vi "Dashboard Main.vi"() -> ()   [LabVIEW 2016]
uses:
  <vilib>/Utility/miscctls.llb/LVRowAndColumnTypeDef.ctl
  <vilib>/event_ctls.llb/eventvkey.ctl
  <vilib>/Rock Robotics/Network Tables/NT Read Numeric Array.vi
  <vilib>/Rock Robotics/WPI/Dashboard/WPI_DashboardLogging Global.vi
panel:
  in  "Camera Settings Right":T1={"Frame Rate"=30, "Compression"=30, "Size"=1, "DB Camera Config"=FALSE} {"Frame Rate" scale=1.0..30.0; "Compression" scale=100.0..-1.0; "Size" items=["640x480", "320x240", "160x120"]}
  in  "Camera Name Right":string(combo)="No Camera Selection"
  out "Camera Info":cluster{"Mbps LED":bool, "Mbps":dbl, "fps":dbl} {"fps" format="%#.1g"; "Mbps" format="%#.1g"}
  in  "Camera Settings":T1={"Frame Rate"=30, "Compression"=30, "Size"=1, "DB Camera Config"=FALSE} {"Frame Rate" scale=1.0..30.0; "Compression" scale=100.0..-1.0; "Size" items=["640x480", "320x240", "160x120"]}
  in  "TCP":refnum<k5>
  in  "Rec Mode":enum32{"Stop", "Record", "Playback"}(radio)
  out "Robot IP":string
  out "Image Message":string="Timeout in Camera Communications"
  in  "Dashboard Tab":T2(tab)
  in  "Select Auto":string(combo)="Select Autonomous ..."
  out "NT Connection":bool
  out "MotorChart R":cluster{"Numeric":dbl, "Numeric":dbl}(graph)
  out "MotorChart L":cluster{"Numeric":dbl, "Numeric":dbl}(graph)
  out "MotorSliders R":cluster{"MotorSlide1":dbl, "MotorSlide2":dbl} {"MotorSlide2" scale=-1.0..1.0 scale format="%#_2e"; "MotorSlide1" scale=-1.0..1.0 scale format="%#_2e"}
  out "MotorSliders L":cluster{"MotorSlide1":dbl, "MotorSlide2":dbl} {"MotorSlide2" scale=-1.0..1.0 scale format="%#_2e"; "MotorSlide1" scale=-1.0..1.0 scale format="%#_2e"}
  out "Gyro":dbl(knob) scale=0.0..360.0
  out "JS1 Z":dbl(slide) scale=-1.0..1.0 scale format="%#_2e"
  out "JS1 Graph":cluster{"X":dbl, "Y":dbl}[](graph)
  out "JS1 Buttons":T3
  out "JS2 Z":dbl(slide) scale=-1.0..1.0 scale format="%#_2e"
  out "JS2 Graph":cluster{"X":dbl, "Y":dbl}[](graph)
  out "JS2 Buttons":T3
  out "Mode":T4(ring)=enum."Auto Disabled"
  out "Camera Image Right":T5(plugin-control)
  in  "DB/String 9":string
  in  "DB/String 8":string
  in  "DB/String 7":string
  in  "DB/String 6":string
  in  "DB/String 5":string
  in  "DB/String 4":string
  in  "DB/String 3":string
  in  "DB/String 2":string
  in  "DB/String 1":string
  in  "DB/String 0":string
  in  "DB/Slider 0":dbl(slide) scale=0.0..5.0
  in  "DB/Slider 1":dbl(slide) scale=0.0..5.0
  in  "DB/Slider 2":dbl(slide) scale=0.0..5.0
  in  "DB/Slider 3":dbl(slide) scale=0.0..5.0
  out "DB/LED 3":bool
  out "DB/LED 2":bool
  out "DB/LED 1":bool
  out "DB/LED 0":bool
  in  "DB/Button 3":bool
  in  "DB/Button 2":bool
  in  "DB/Button 1":bool
  in  "DB/Button 0":bool caption="New Name"
  out "Right Speed":cluster{dbl, dbl}(knob) scale=0.0..3500.0
  out "Left Speed":cluster{dbl, dbl}(knob)={0.0, 1631.277968125847} scale=0.0..3500.0
  out "Right Throttle":dbl
  out "Right Current":dbl
  out "Left Throttle":dbl
  out "Left Current":dbl
  out "Power Consumed":dbl
  out "Voltage":dbl(knob) scale=0.0..14.0
  out "Current Draw":dbl(knob) scale=0.0..300.0
  in  "OSC Stream":bool
  in  "Test Slider":dbl(slide) scale=0.0..100.0 scale format="%#_3g"
  in  "On/Off":bool caption="Solenoid"
  in  "Test Name":u16(ring) items=["Select the test to run..."]
  in  "Test Tree":string(tree)
  in  "Motor":cluster{"Value":dbl, "Enable":bool} {"Value" scale=-1.0..1.0 scale format="%#_3g"}
  out "Progress":T6 {"Test Progress" scale=0.0..100.0}
  in  "Rev/Fwd":cluster{"Forward":bool, "Reverse":bool}
  in  "Test Ring":u16(ring) items=["Monochrome", "Color"]
  out "Cmd Status":string
  in  "Execute Command":bool
  in  "Command Params":string[][](table)
  in  "Command Selection":i32(listbox)
  in  "CheckList":i32(listbox)
  out "Tree":string(tree)
  out "Camera Image":T5(plugin-control)
  out "Background":bool
  in  "Camera Name":string(combo)="No Camera Selection"
  # "HW"
  # "HW"
  # "Joysticks"
  # "Drive Motors"
  # "Front"
  # "Right"
  # "Left"
  # "Back"
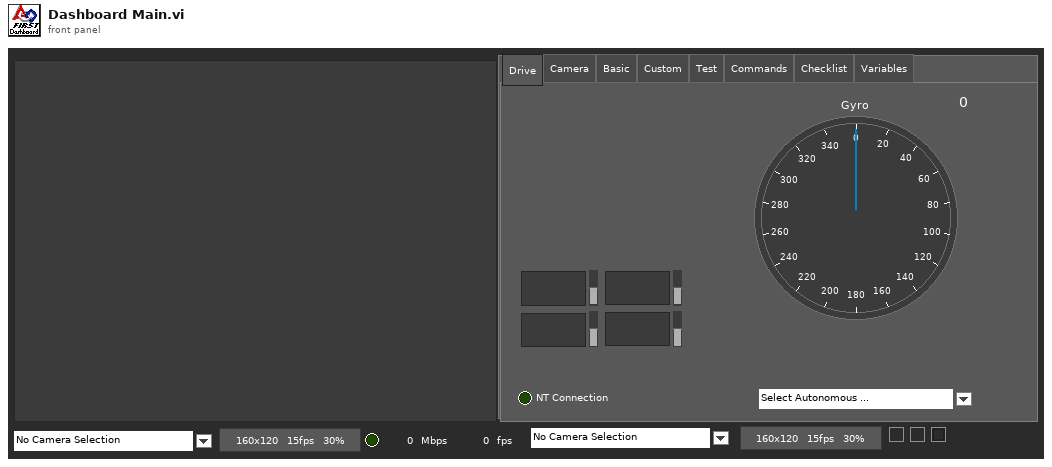
[diagram p1: front panel]
types:
  T1 = cluster{"Frame Rate":i32, "Compression":i32, "Size":u16, "DB Camera Config":bool}
  T2 = enum32{"Drive", "Camera", "Basic", "Custom", "Test", "Commands", "Checklist", "Variables"}
  T3 = cluster{bool, bool, bool, bool, bool, bool, bool, bool, bool, bool, bool, bool}
  T4 = enum8{"Tele-Op Disabled", "Tele-Op Enabled", "Auto Disabled", "Auto Enabled", "Test Disabled", "Test Enabled", "Disconnected", "No Code", "E-Stop"}
  T5 = typedef "IMAQ Image.ctl" = refnum<image>
  T6 = cluster{"Test Progress":u8, "Test Progress Text":string}
  T7 = typedef "Image Type" = u32
  T8 = cluster{"IDs":cluster{"RPC field ID":u16, "Unique ID":u16}, "String":string}
  T9 = enum32{"Drive", "Basic", "Custom", "Test", "Checklist", "Variables"}
  T10 = cluster{"Error Strings":string, "Disable Counts":cluster{u16, u16}, "Rail Faults":cluster{u16, u16, u16}, "Robot IP":string, "DB Mode":u8, "Event Info":cluster{"Name":string, "Type":u8, "Number":u16, "Replay":u8}}
  T11 = cluster{"Storage":cluster{"Disk Free":u64, "RAM Block":u32, "RAM free":u32}, "CPU Utilization":cluster{"CPU % ISR":sgl, "CPU % Time Crit":sgl, "CPU % Timed Str":sgl, "CPU % High":sgl, "CPU % Above":sgl, "CPU % Normal":sgl, "CPU % Low":sgl}, "CAN":cluster{"% Bus Utilization":sgl, "Bus Off Cnt":u32, "TX_FIFO Full Cnt":u32, "Receive Error Cnt":u8, "Transmit Error Cnt":u8}, "HID":cluster{"HID Outputs":u32, "Rumble Low":u16, "Rumble High":u16}[]}
  T12 = cluster{"Status bits":cluster{"Test Mode":bool, "Autonomous":bool, "Enabled":bool, "Code Start":bool, "Brownout":bool, "Reserved 2":bool, "Reserved 3":bool, "E-Stop":bool}, "Code Trace":cluster{"Disabled":bool, "TeleOp":bool, "Auto":bool, "Test":bool}, "Controller Type":enum16{"unknown", "cRIO", "roboRio"}, "Code?":enum16{"unknown", "noCode", "code"}, "Battery V":dbl}
  T13 = cluster{"Control Bits":cluster{"TestMode":bool, "Autonomous":bool, "Enabled":bool, "FMS Present":bool, bool, bool, bool, "E-Stop":bool}, "Team Station ":u8, "Countdown":sgl, "Joystick Values":cluster{"Axes":dbl[], "Buttons":bool[], "POVs":i16[]}[]}
  T14 = cluster{"Axes":dbl[], "Buttons":bool[], "POVs":i16[]}[]
  T15 = cluster{"Axes":dbl[], "Buttons":bool[], "POVs":i16[]}
  T16 = cluster{"Buttons[0]":bool, "Buttons[1]":bool, "Buttons[2]":bool, "Buttons[3]":bool, "Buttons[4]":bool, "Buttons[5]":bool, "Buttons[6]":bool, "Buttons[7]":bool, "Buttons[8]":bool, "Buttons[9]":bool, "Buttons[10]":bool, "Buttons[11]":bool}
  T17 = cluster{"Camera Image":refnum<vi>, "Dashboard Tab":refnum<vi>, "Background":refnum<vi>, "Rec Mode":refnum<vi>, "Test Slider":refnum<vi>, "On/Off ":refnum<vi>, "Test Ring":refnum<vi>, "Rev/Fwd":refnum<vi>, "Test Name":refnum<vi>, "Motor":refnum<vi>, "Progress":refnum<vi>, "CheckList":refnum<vi>, "Tree":refnum<vi>, "Test Tree":refnum<vi>, "Command Params":refnum<vi>, "Command Selection":refnum<vi>, "Execute Command":refnum<vi>, "Cmd Status":refnum<vi>, "Camera Settings":refnum<vi>, "Camera Name":refnum<vi>, "Camera Info":refnum<vi>, "Camera Settings Right":refnum<vi>, "Camera Name Right":refnum<vi>, "Camera Image Right":refnum<vi>}
  T18 = cluster{"Operation":enum16{"Update", "Clear"}, "Color Box":u32}[]
  T19 = typedef "eventvkey.ctl" = enum16{"ASCII", "Enter", "Return", "Shift", "Ctrl", "Alt", "Cmd", "Opt", "Caps", "NumLock", "Clear", "Break", "Up", "Down", "Left", "Right", "Insert", "Delete", "Home", "End", "PageUp", "PageDown", "Escape", "Help", "Pause", "ScrollLock", "F1", "F2", "F3", "F4", "F5", "F6", "F7", "F8", "F9", "F10", "F11", "F12", "F13", "F14", "F15", "F16", "F17", "F18", "F19", "F20", "F21", "F22", "F23", "F24", "Play", "VolumeUp", "VolumeDown", "Mute", "Two Byte Char"}
  T20 = cluster{"Image Size":bool, "Image Type":bool, "Pixel Value":bool, "ROI Information":bool, "Zoom Factor":bool}
  T21 = cluster{"Operation":enum16{"Update", "Clear"}, "Color Box":u32}
  T22 = typedef "LVRowAndColumnTypeDef.ctl" = cluster{"Row":i32, "Column":i32}
  T23 = cluster{"Shift":bool, "Ctrl":bool, "Alt":bool, "Cmd":bool, "Opt":bool}
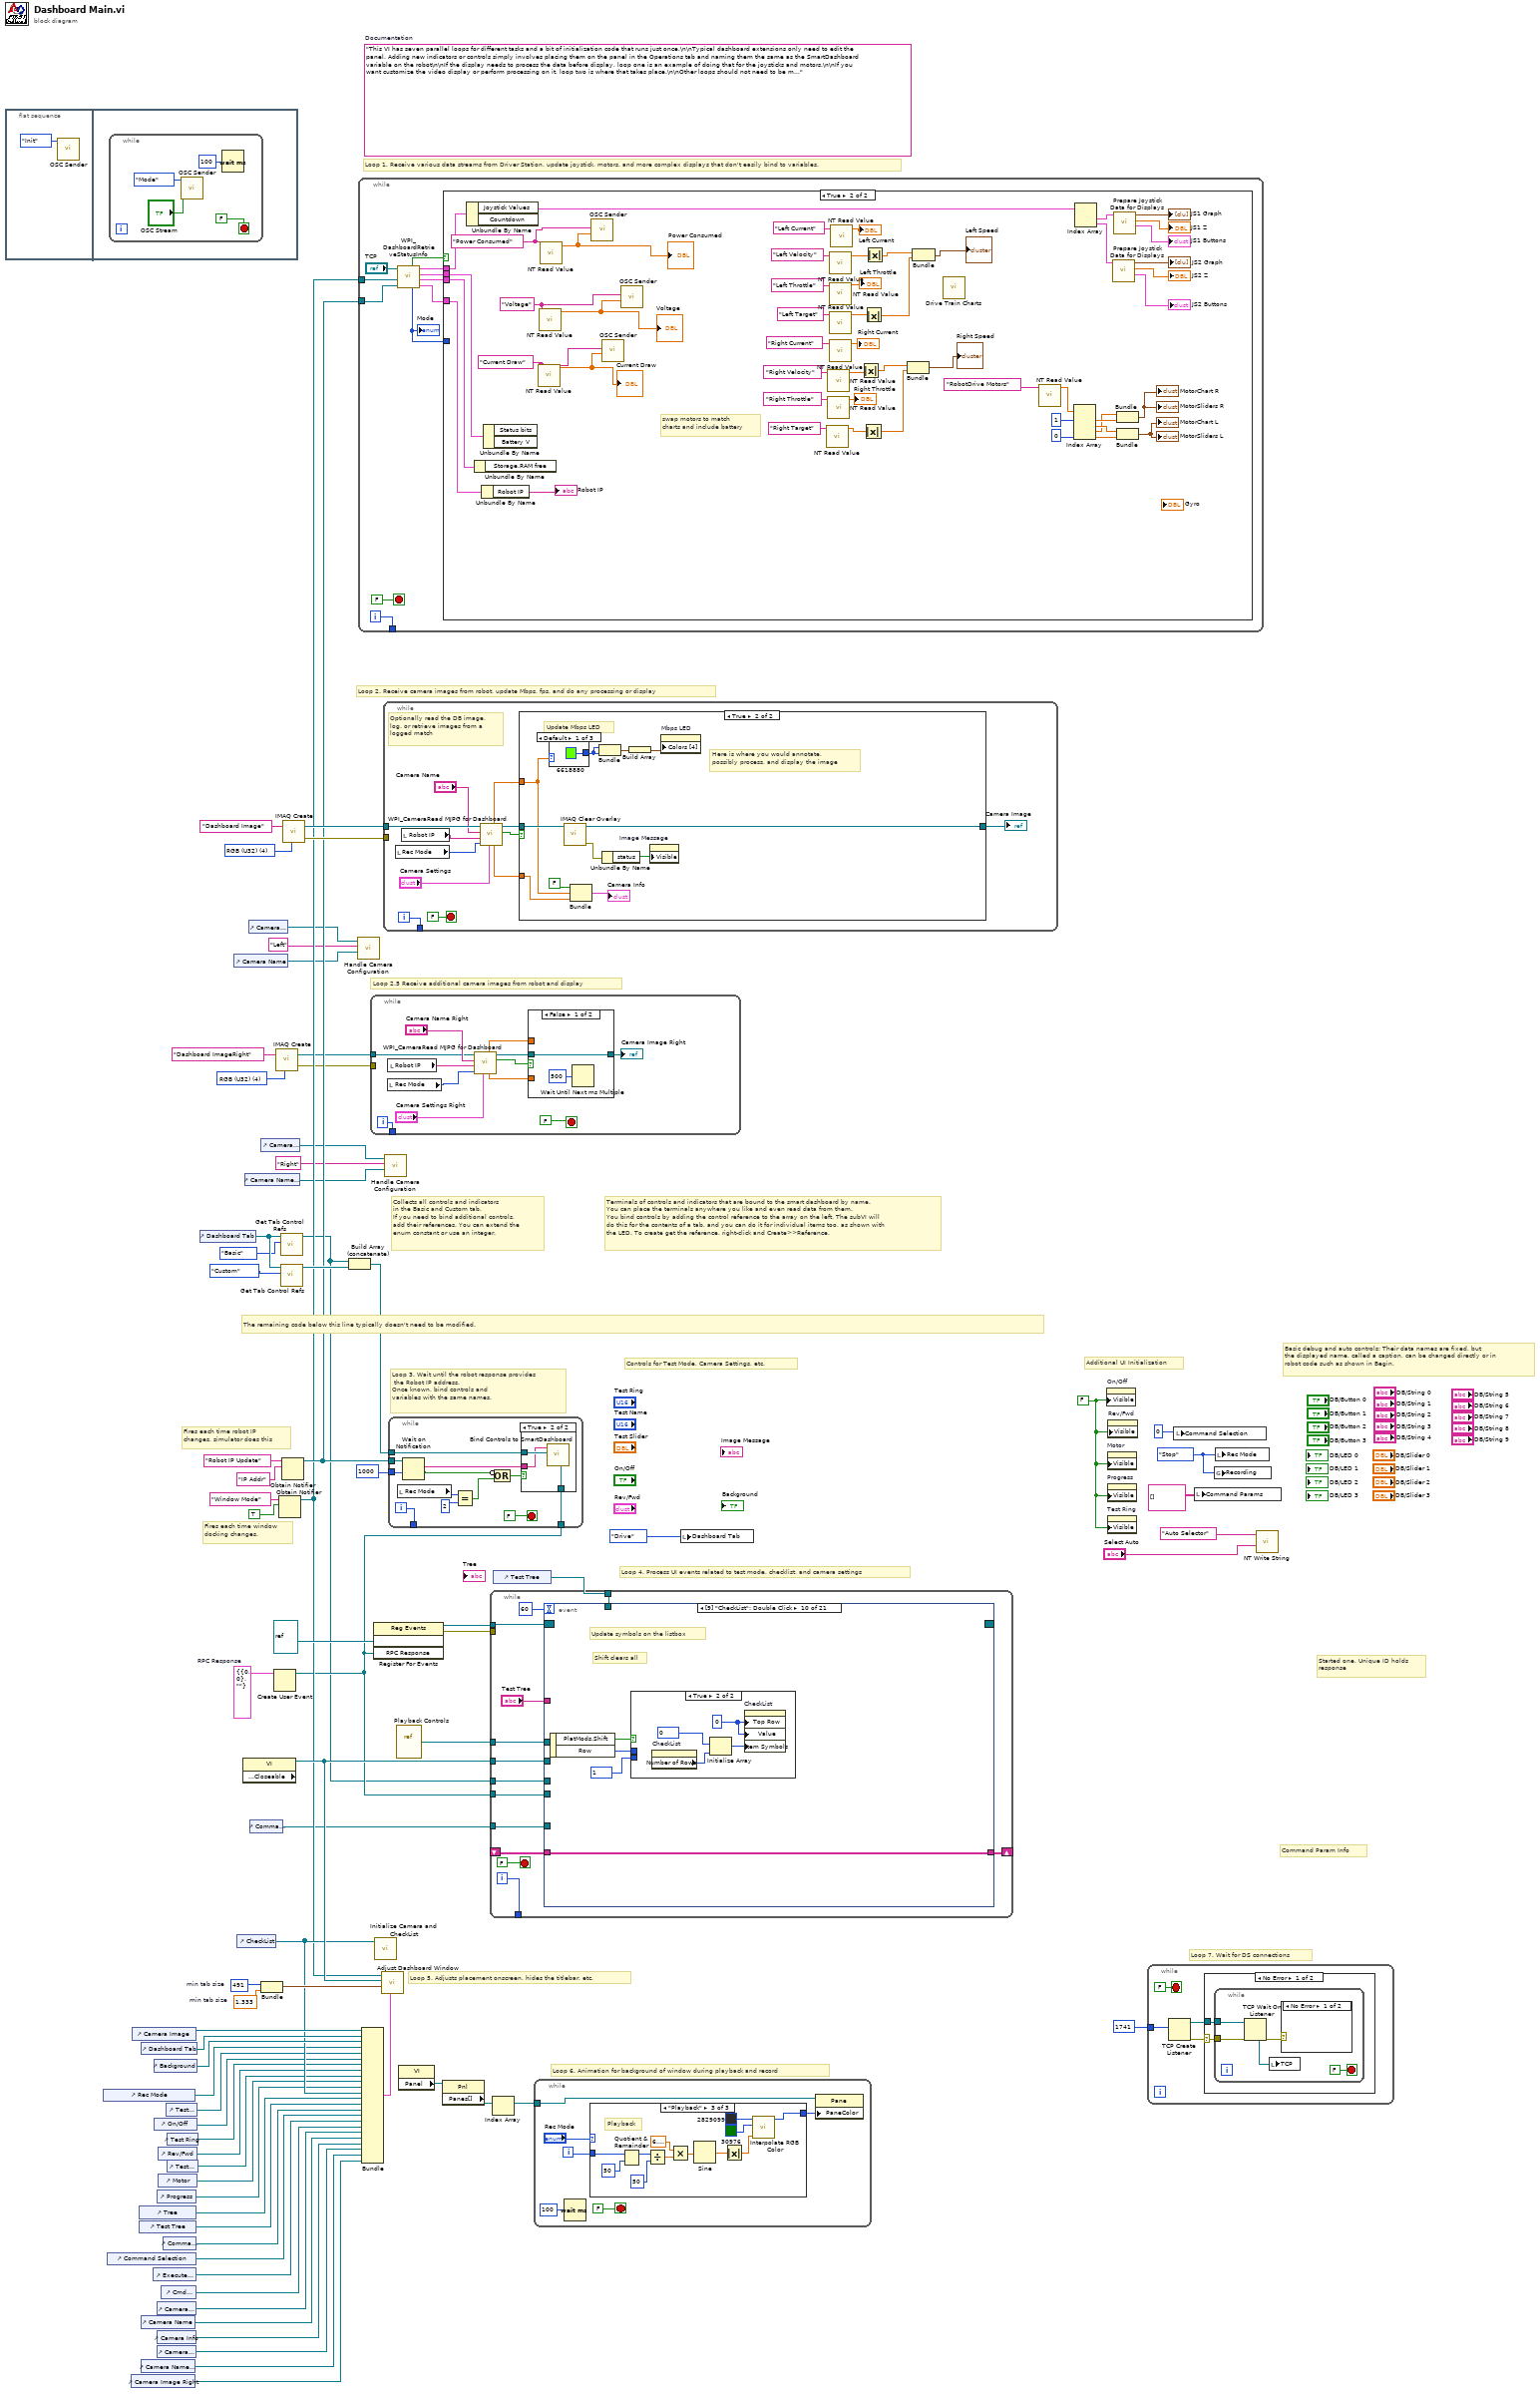
[diagram p0: block diagram]
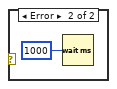
[diagram p3: hidden frame]
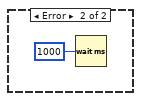
[diagram p4: hidden frame]
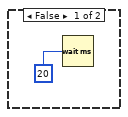
[diagram p5: hidden frame]
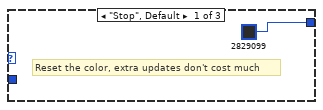
[diagram p6: hidden frame]
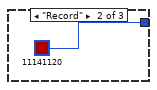
[diagram p7: hidden frame]
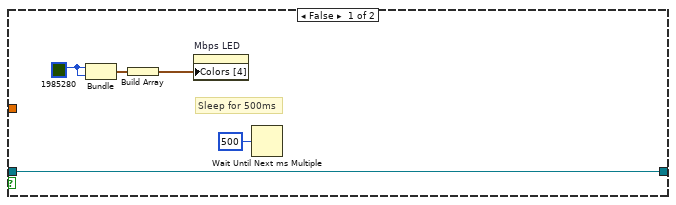
[diagram p9: hidden frame]
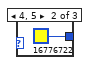
[diagram p10: hidden frame]
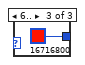
[diagram p11: hidden frame]
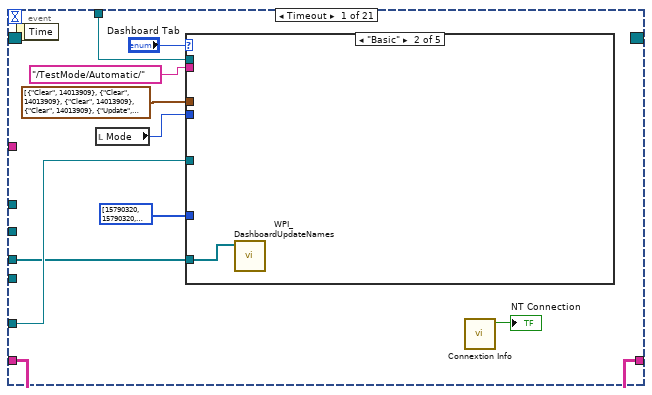
[diagram p12: hidden frame]
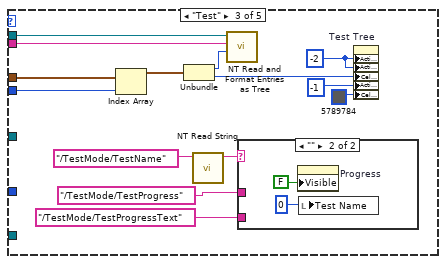
[diagram p14: hidden frame]
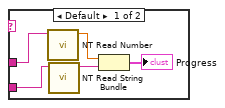
[diagram p15: hidden frame]
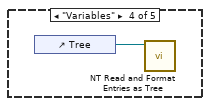
[diagram p16: hidden frame]
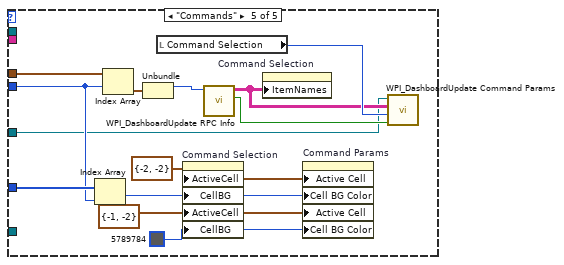
[diagram p17: hidden frame]
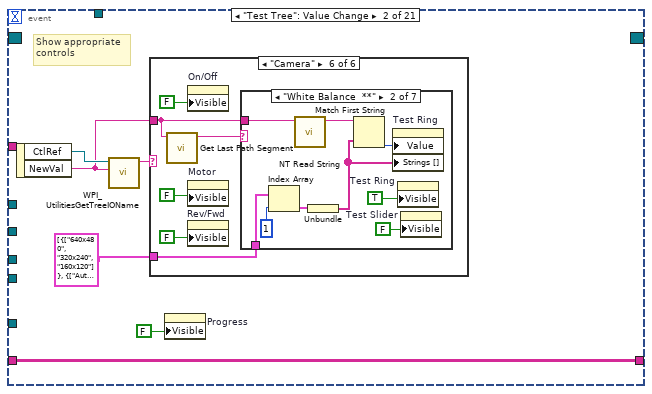
[diagram p18: hidden frame]
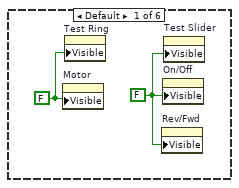
[diagram p19: hidden frame]
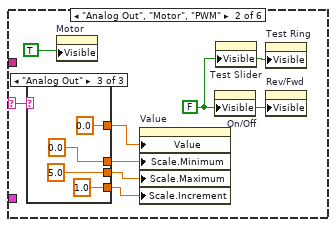
[diagram p20: hidden frame]
diagram:
  w10 = T7 4 items=["Grayscale (U8)", "Grayscale (I16)", "Grayscale (SGL)", "Complex (CSG)", "RGB (U32)", "HSL (U32)", "RGB (U64)"] ("Image Type")
  w26 = T8 {"IDs"={"RPC field ID"=0, "Unique ID"=0}, "String"=""}  # RPC Response
  w51 = 491  # min tab size
  w50 = 1.333  # min tab size
  w58 = enum32{"Stop", "Record", "Playback"}."Stop" ("Rec Mode")
  w33 = FALSE ("Visible")
  (unwired) "This VI has seven parallel loops for different tasks and a bit of initialization code that runs just once.\n\nTypical dashboard extensions only need to edit the panel. Adding new indicators or controls simply involves placing them on the panel in the Operations tab and naming them the same as the SmartDashboard variable on the robot\n\nIf the display needs to process the data before display, loop one is an example of doing that for the joysticks and motors.\n\nIf you want customize the video display or perform processing on it, loop two is where that takes place.\n\nOther loops should not need to be modified. They are pretty standard, and document the task they perform."  # Documentation
  w75 = T7 4 items=["Grayscale (U8)", "Grayscale (I16)", "Grayscale (SGL)", "Complex (CSG)", "RGB (U32)", "HSL (U32)", "RGB (U64)"] ("Image Type")
  # "Loop 2.5 Receive additional camera images from robot and display"
  # "Command Param Info"
  # "Started one, Unique ID holds\nresponse"
  # "Loop 7. Wait for DS connections"
  # "Basic debug and auto controls: Their data names are fixed, but\nthe displayed name, called a caption, can be changed directly or in\nrobot code such as shown in Begin."
  # "Controls for Test Mode, Camera Settings, etc."
  # "Additional UI Initialization"
  # "Loop 6. Animation for background of window during playback and record"
  # "Fires each time robot IP\nchanges, simulator does this"
  # "Fires each time window\ndocking changes."
  # "Collects all controls and indicators\nin the Basic and Custom tab.\nIf you need to bind additional controls,\nadd their references. You can extend the\nenum constant or use an integer."
  # "The remaining code below this line typically doesn't need to be modified."
  # "Loop 4. Process UI events related to test mode, checklist, and camera settings"
  # "Terminals of controls and indicators that are bound to the smart dashboard by name.\nYou can place the terminals anywhere you like and even read data from them.\nYou bind controls by adding the control reference to the array on the left. The subVI will\ndo this for the contents of a tab, and you can do it for individual items too, as shown with\nthe LED. To create get the reference, right-click and Create>>Reference."
  # "Loop 3. Wait until the robot response provides\n the Robot IP address.\nOnce known, bind controls and\nvariables with the same names."
  # "Loop 5. Adjusts placement onscreen, hides the titlebar, etc."
  # "Loop 1. Receive various data streams from Driver Station, update joystick, motors, and more complex displays that don't easily bind to variables."
  # "Loop 2. Receive camera images from robot, update Mbps, fps, and do any processing or display"
  n1 = flat-sequence {
    frame #0 {
      n2 = call "OSC Sender.vi"("State"=enum16{"Init", "Send", "Mode"}."Init") -> ()  [unwired: 11 in]
    }
    frame #1 {
      n3 = while {
        stop <- FALSE stop-if-true
        n4 = call "OSC Sender.vi"("Mode"="OSC Stream", "State"=enum16{"Init", "Send", "Mode"}."Mode") -> ()  [unwired: 10 in]
        n5 = Wait (ms)(milliseconds to wait=u32 100) -> ()  [unwired: 1 out]
      }
    }
  }
  n6 = control-ref of="Rec Mode"() -> (w39:refnum<vi>)
  n7 = control-ref of="Command Selection"() -> (w25:refnum<vi>)
  n8 = control-ref of="Camera Image Right"() -> (w1:refnum<vi>)
  n9 = control-ref of="Camera Image"() -> (w53:refnum<vi>)
  n10 = control-ref of="Tree"() -> (w43:refnum<vi>)
  n11 = control-ref of="Test Tree"() -> (w42:refnum<vi>)
  n12 = control-ref of="Dashboard Tab"() -> (w52:refnum<vi>)
  n13 = control-ref of="Camera Name"() -> (w16:refnum<vi>)
  n14 = control-ref of="Camera Name Right"() -> (w2:refnum<vi>)
  n15 = control-ref of="Execute Command"() -> (w27:refnum<vi>)
  n16 = control-ref of="Background"() -> (w48:refnum<vi>)
  n17 = control-ref of="On/Off"() -> (w37:refnum<vi>)
  n18 = control-ref of="Progress"() -> (w34:refnum<vi>)
  n19 = control-ref of="Camera Settings"() -> (w17:refnum<vi>)
  n20 = control-ref of="Camera Info"() -> (w15:refnum<vi>)
  n21 = control-ref of="Camera Settings Right"() -> (w3:refnum<vi>)
  n22 = control-ref of="Rev/Fwd"() -> (w35:refnum<vi>)
  n23 = control-ref of="Motor"() -> (w40:refnum<vi>)
  n24 = control-ref of="Cmd Status"() -> (w21:refnum<vi>)
  n25 = control-ref of="Command Params"() -> (w28:refnum<vi>)
  n26 = control-ref of="Test Slider"() -> (w38:refnum<vi>)
  n27 = control-ref of="Test Ring"() -> (w36:refnum<vi>)
  n28 = control-ref of="Test Name"() -> (w41:refnum<vi>)
  n29 = control-ref of="Dashboard Tab"() -> (w56:refnum<vi>)
  n30 = control-ref of="Camera Name"() -> (w18:refnum<vi>)
  n31 = control-ref of="CheckList"() -> (w44:refnum<vi>)
  n32 = property class="VI" props=["Front Panel.Closeable"]() -> (reference out=w57:refnum<vi>)  [unwired: 2 in, 2 out]
  n33 = control-ref of="Camera Name Right"() -> (w6:refnum<vi>)
  n34 = control-ref of="Camera Settings"() -> (w19:refnum<vi>)
  n35 = control-ref of="Command Params"() -> (w20:refnum<vi>)
  n36 = control-ref of="Camera Settings Right"() -> (w7:refnum<vi>)
  n37 = Bundle("min tab size"=w51, "min tab size"=w50) -> (w49:cluster{"min tab size":i32, "min tab size":dbl})  [unwired: 1 in]
  n38 = Create User Event(user event datatype=w26) -> (user event=w22:refnum<user-event>)  [unwired: 1 in, 1 out]
  n39 = call "IMAQ Create"("Image Name"="Dashboard ImageRight", "Image Type"=w10) -> ("New Image"=w9:T5, "error out"=w8:errorcluster)  [unwired: 2 in, 1 out]
  n40 = Obtain Notifier(name (unnamed)="Window Mode", notification data type=TRUE) -> (notifier out=w31:refnum<notifier>)  [unwired: 2 in, 2 out]
  n41 = call <vilib>:"Get Tab Control Refs.vi"("Page Index"=T9."Basic" ("Dashboard Tab"), "TabControl in"=w56) -> ("ControlsOnPage"=w14:refnum<vi>[])  [unwired: 9 in]
  n42 = call <vilib>:"Get Tab Control Refs.vi"("Page Index"=T9."Custom" ("Dashboard Tab"), "TabControl in"=w56) -> ("ControlsOnPage"=w55:refnum<vi>[])  [unwired: 9 in]
  n43 = Obtain Notifier(name (unnamed)="Robot IP Update", notification data type="IP Addr" ("name (unnamed)")) -> (notifier out=w32:refnum<notifier>)  [unwired: 2 in, 2 out]
  n44 = call "IMAQ Create"("Image Name"="Dashboard Image", "Image Type"=w75) -> ("New Image"=w73:T5, "error out"=w72:errorcluster)  [unwired: 2 in, 1 out]
  n45 = Build Array (concatenate)(w14, w55) -> (w54:refnum<vi>[])
  n46 = call "Handle Camera Configuration.vi"("CameraNameRef"=w18, "Camera File Name"="Left", "ClusterRef"=w19) -> ()  [unwired: 9 in]
  n47 = while {
    tunnel: [w90] -> _
    tunnel: w32 -> [w84]
    tunnel: w31 -> [w81]
    i -> [w90]
    stop <- FALSE stop-if-true
    n48 = call <vilib>:"WPI_DashboardRetrieveStatusInfo.vi"("Binding Refnum"=w84, "Window Mode Notifier"=w81, "TCP Cnx"="TCP") -> ("Power and Errors"=w85:T10, "Robot Metrics"=w88:T11, "Status Info"=w89:T12, "Control Info"=w86:T13, "Robot Mode"=w83:T4, "Process?"=w87:bool)  [unwired: 3 in]
    "Mode" <- w83
    n49 = case shown="True" w87 {
      tunnel: w89 -> [_ w144]
      tunnel: w88 -> [_ w143]
      tunnel: w86 -> [_ w142]
      tunnel: w85 -> [_ w141]
      tunnel: w83 -> [_ _]
      frame False {
        n50 = Wait (ms)(milliseconds to wait=u32 20) -> ()  [unwired: 1 out]
      }
      frame True {
        w94 = "Current Draw" ("Name")
        w96 = "Voltage" ("Name")
        w98 = "Power Consumed" ("Name")
        # "swap motors to match\ncharts and include battery"
        n51 = Unbundle By Name(w142) -> ("Joystick Values"=w132:T14)  [unwired: 1 out]
        n52 = Unbundle By Name(w143) -> ()  [unwired: 1 out]
        n53 = Unbundle By Name(w141) -> ("Robot IP"=→"Robot IP":string)
        n54 = Unbundle By Name(w144) -> ()  [unwired: 2 out]
        n55 = call-poly <vilib>:"NT Read Value.vi"("Name"=w94) -> ("Numeric"=w93:dbl)  [unwired: 9 in, 1 out]
        "Current Draw" <- w93
        n56 = call-poly <vilib>:"NT Read Value.vi"("Name"=w96) -> ("Numeric"=w95:dbl)  [unwired: 9 in, 1 out]
        "Voltage" <- w95
        n57 = call-poly <vilib>:"NT Read Value.vi"("Name"=w98) -> ("Numeric"=w97:dbl)  [unwired: 9 in, 1 out]
        "Power Consumed" <- w97
        n58 = call "OSC Sender.vi"("Value"=w97, "Label"=w98) -> ()  [unwired: 10 in]
        n59 = call "OSC Sender.vi"("Value"=w93, "Label"=w94) -> ()  [unwired: 10 in]
        n60 = call "OSC Sender.vi"("Value"=w95, "Label"=w96) -> ()  [unwired: 10 in]
        n61 = call-poly <vilib>:"NT Read Value.vi"("Name"="Right Target") -> ("Numeric"=w107:dbl)  [unwired: 9 in, 1 out]
        n62 = call-poly <vilib>:"NT Read Value.vi"("Name"="Right Velocity") -> ("Numeric"=w106:dbl)  [unwired: 9 in, 1 out]
        n63 = call-poly <vilib>:"NT Read Value.vi"("Name"="Right Throttle") -> ("Numeric"=→"Right Throttle":dbl)  [unwired: 9 in, 1 out]
        n64 = call-poly <vilib>:"NT Read Value.vi"("Name"="Right Current") -> ("Numeric"=→"Right Current":dbl)  [unwired: 9 in, 1 out]
        n65 = call-poly <vilib>:"NT Read Value.vi"("Name"="Left Velocity") -> ("Numeric"=w108:dbl)  [unwired: 9 in, 1 out]
        n66 = call-poly <vilib>:"NT Read Value.vi"("Name"="Left Throttle") -> ("Numeric"=→"Left Throttle":dbl)  [unwired: 9 in, 1 out]
        n67 = call-poly <vilib>:"NT Read Value.vi"("Name"="Left Target") -> ("Numeric"=w105:dbl)  [unwired: 9 in, 1 out]
        n68 = call-poly <vilib>:"NT Read Value.vi"("Name"="Left Current") -> ("Numeric"=→"Left Current":dbl)  [unwired: 9 in, 1 out]
        n69 = Absolute Value(x=w106) -> (abs(x)=w102:dbl)
        n70 = Absolute Value(x=w107) -> (abs(x)=w101:dbl)
        n71 = Absolute Value(x=w105) -> (abs(x)=w103:dbl)
        n72 = Absolute Value(x=w108) -> (abs(x)=w104:dbl)
        n73 = Bundle(w102, w101) -> (→"Right Speed":cluster{dbl, dbl})  [unwired: 1 in]
        n74 = Bundle(w104, w103) -> (→"Left Speed":cluster{dbl, dbl})  [unwired: 1 in]
        n75 = call "Drive Train Charts.vi"() -> ()  [unwired: 12 in]
        n76 = call-poly <vilib>:"NT Read Value.vi"("Name"="RobotDrive Motors") -> ("Numeric Array"=w122:dbl[])  [unwired: 9 in, 1 out]
        n77 = Index Array(array=w122, index #1=1, index #4=0) -> (element #1=w136:dbl, element #2=w137:dbl, element #3=w135:dbl, element #4=w140:dbl)  [unwired: 2 in]
        n78 = Index Array(array=w132) -> (element #1=w131:T15, element #2=w127:T15)  [unwired: 2 in]
        n79 = call "Prepare Joystick Data for Displays.vi"("Joystick Values"=w127) -> ("Buttons"=→"JS2 Buttons":T16, "Z Axis"=→"JS2 Z":dbl, "Cartesian Data"=→"JS2 Graph":cluster{"X axis":dbl, "X axis":dbl}[])  [unwired: 8 in]
        n80 = call "Prepare Joystick Data for Displays.vi"("Joystick Values"=w131) -> ("Buttons"=→"JS1 Buttons":T16, "Z Axis"=→"JS1 Z":dbl, "Cartesian Data"=→"JS1 Graph":cluster{"X axis":dbl, "X axis":dbl}[])  [unwired: 8 in]
        n81 = Bundle("Numeric"=w135, "Numeric"=w136) -> (→"MotorChart R" →"MotorSliders R":cluster{"Numeric":dbl, "Numeric":dbl})  [unwired: 1 in]
        n82 = Bundle("Numeric"=w137, "Numeric"=w140) -> (→"MotorChart L" →"MotorSliders L":cluster{"Numeric":dbl, "Numeric":dbl})  [unwired: 1 in]
      }
    }
  }
  n83 = Bundle("Camera Image"=w53, "Dashboard Tab"=w52, "Background"=w48, "Rec Mode"=w39, "Test Slider"=w38, "On/Off"=w37, "Test Ring"=w36, "Rev/Fwd"=w35, "Test Name"=w41, "Motor"=w40, "Progress"=w34, "CheckList"=w44, "Tree"=w43, "Test Tree"=w42, "Command Params"=w28, "Command Selection"=w25, "Execute Command"=w27, "Cmd Status"=w21, "Camera Settings"=w17, "Camera Name"=w16, "Camera Info"=w15, "Camera Settings Right"=w3, "Camera Name Right"=w2, "Camera Image Right"=w1) -> (w45:T17)  [unwired: 1 in]
  n84 = while {
    tunnel: w9 -> [w155]
    tunnel: w8 -> [_]
    tunnel: [w149] -> _
    i -> [w149]
    stop <- FALSE stop-if-true
    n85 = local read "Rec Mode"() -> (w153:enum32{"Stop", "Record", "Playback"})
    n86 = local read "Robot IP"() -> (w154:string)
    n87 = call <vilib>:"WPI_CameraRead MJPG for Dashboard.vi"("Camera Settings"="Camera Settings Right", "Rec Mode"=w153, "Robot IP"=w154, "Camera Name"="Camera Name Right", "Refnum in"=w155) -> ("Active"=w148:bool, "Refnum out"=w151:T5, "FPS"=w146:dbl, "Bandwidth (Mbps)"=w147:dbl)  [unwired: 3 in]
    n88 = case shown="False" w148 {
      tunnel: w151 -> [w157 w159]
      tunnel: w147 -> [_ _]
      tunnel: w146 -> [_ _]
      tunnel: [w157 w159] -> w145
      frame False {
        n89 = Wait Until Next ms Multiple(millisecond multiple=u32 500) -> ()  [unwired: 1 out]
      }
      frame True {
      }
    }
    "Camera Image Right" <- w145
  }
  n90 = register-events(refnum<vi> refnum, w22) -> (reference out=w62:refnum<event-registration>, error out=w61:errorcluster)  [unwired: 2 in]
  n91 = call "Initialize Camera and CheckList.vi"("ListBox in"=w44) -> ()  [unwired: 11 in]
  n92 = call "Adjust Dashboard Window.vi"("Sizing Refnums"=w45, "Size Constraints"=w49, "VI"=w57, "WIn Mode"=w31) -> ()  [unwired: 8 in]
  n93 = while {
    tunnel: w73 -> [w169]
    tunnel: w72 -> [_]
    tunnel: [w170] -> _
    i -> [w170]
    stop <- FALSE stop-if-true
    # "Optionally read the DB image,\nlog, or retrieve images from a\nlogged match"
    n94 = local read "Rec Mode"() -> (w165:enum32{"Stop", "Record", "Playback"})
    n95 = local read "Robot IP"() -> (w164:string)
    n96 = call <vilib>:"WPI_CameraRead MJPG for Dashboard.vi"("Camera Settings"="Camera Settings", "Rec Mode"=w165, "Robot IP"=w164, "Camera Name"="Camera Name", "Refnum in"=w169) -> ("Active"=w167:bool, "Refnum out"=w168:T5, "FPS"=w166:dbl, "Bandwidth (Mbps)"=w163:dbl)  [unwired: 3 in]
    n97 = case shown="True" w167 {
      tunnel: w168 -> [w172 w183]
      tunnel: w163 -> [_ w180]
      tunnel: w166 -> [_ w181]
      tunnel: [w172 w177] -> w160
      frame False {
        w174 = u32 1985280 ("Color Box")
        # "Sleep for 500ms"
        n98 = Bundle("Color Box"=w174, "Color Box"=w174) -> (w175:cluster{"Color Box":u32, "Color Box":u32})  [unwired: 1 out]
        n99 = Build Array(w175) -> (w173:cluster{"Color Box":u32, "Color Box":u32}[])
        n100 = property on="Mbps LED" class="Bool (strict)"("Colors [4]"=w173) -> ()  [unwired: 2 in, 2 out]
        n101 = Wait Until Next ms Multiple(millisecond multiple=u32 500) -> ()  [unwired: 1 out]
      }
      frame True {
        # "Here is where you would annotate,\npossibly process, and display the image"
        # "Update Mbps LED"
        n102 = case shown="Default" w180 {
          tunnel: [u32 6618880 ("Color Box") u32 16776722 ("Color Box") u32 16716800 ("Color Box")] -> w184
          frame Default {
          }
          frame 4, 5 {
          }
          frame 6.. {
          }
        }
        n103 = call "IMAQ Clear Overlay"("Image"=w183) -> ("error out"=w186:errorcluster, "Image Out"=w177:T5)  [unwired: 2 in, 7 out]
        n104 = Bundle(FALSE, "Bandwidth (Mbps)"=w180, "FPS"=w181) -> (→"Camera Info":cluster{bool, "Bandwidth (Mbps)":dbl, "FPS":dbl})  [unwired: 1 in]
        n105 = Bundle("Color Box"=w184, "Color Box"=w184) -> (w185:cluster{"Color Box":u32, "Color Box":u32})  [unwired: 1 out]
        n106 = Unbundle By Name(w186) -> ("status"=w187:bool)
        n107 = Build Array(w185) -> (w182:cluster{"Color Box":u32, "Color Box":u32}[])
        n108 = property on="Image Message" class="Str"("Visible"=w187) -> ()  [unwired: 2 in, 2 out]
        n109 = property on="Mbps LED" class="Bool (strict)"("Colors [4]"=w182) -> ()  [unwired: 2 in, 2 out]
      }
    }
    "Camera Image" <- w160
  }
  n110 = call "Handle Camera Configuration.vi"("CameraNameRef"=w6, "Camera File Name"="Right", "ClusterRef"=w7) -> ()  [unwired: 9 in]
  n111 = while {
    tunnel: w54 -> [w202]
    tunnel: w32 -> [w200]
    tunnel: [w198] -> _
    tunnel: u32 1000 ("milliseconds to wait") -> [w197]
    tunnel: w22 -> [w191]
    i -> [w198]
    stop <- FALSE stop-if-true
    n112 = local read "Rec Mode"() -> (w193:enum32{"Stop", "Record", "Playback"})
    n113 = Wait on Notification(notifier=w200, timeout in ms (-1)=w197) -> (notification=w199:string, timed out?=w195:bool)  [unwired: 2 in, 2 out]
    n114 = Equal?(x=w193, y=u16 2 ("Rec Mode")) -> (x = y?=w194:bool)
    n115 = Compound Arithmetic op=OR(invert w195, w194) -> (w196:bool)
    n116 = case shown="True" w196 {
      tunnel: w202 -> [_ w205]
      tunnel: w199 -> [_ w204]
      tunnel: w191 -> [_ w203]
      frame False {
      }
      frame True {
        n117 = call <vilib>:"Bind Controls to SmartDashboard.vi"("RPC ref"=w203, "Bound Control Refs"=w205, "Server IP Address"=w204) -> ()  [unwired: 9 in]
      }
    }
  }
  n118 = vi-ref "Playback Controls.vi"() -> (w63:refnum<vi>)
  n119 = property class="VI"() -> ("Panel"=w65:refnum<vi>)  [unwired: 2 in, 2 out]
  n120 = property class="Pnl"(reference=w65) -> ("Panes[]"=w66:refnum<vi>[])  [unwired: 1 in, 2 out]
  n121 = Index Array(array=w66) -> (element=w64:refnum<vi>)  [unwired: 1 in]
  n122 = control-ref of="Test Tree"() -> (w67:refnum<vi>)
  n123 = while {
    tunnel: [w215] -> _
    tunnel: w67 -> [w214]
    tunnel: w63 -> [w213]
    tunnel: w62 -> [w212]
    tunnel: w61 -> [_]
    tunnel: w57 -> [w211]
    tunnel: w22 -> [w210]
    tunnel: w20 -> [w209]
    shift-right: [w208] -> _
    shift-left: _ -> [w207]
    tunnel: w14 -> [w206]
    i -> [w215]
    stop <- FALSE stop-if-true
    n124 = event shown="[9] \"CheckList\": Double Click" {
      selector: w212 -> [_ _ _ _ _ _ _ _ _ _ _ _ _ _ _ _ _ _ _ _ _]
      dyn-events: [_ _ _ _ _ _ _ _ _ _ _ _ _ _ _ _ w471 _ _ _ _] -> _
      timeout: u32 60 ("milliseconds to wait") -> [_ _ _ _ _ _ _ _ _ _ _ _ _ _ _ _ _ _ _ _ _]
      tunnel: w214 -> [w227 _ _ _ _ _ _ _ _ _ _ _ _ _ _ _ _ _ _ _ _]
      tunnel: "Test Tree" -> [_ _ _ _ _ _ _ _ _ _ _ w438 w446 w448 w452 w460 _ _ _ _ _]
      tunnel: w213 -> [_ _ _ _ _ _ _ _ _ _ _ _ _ _ _ _ w473 _ w491 _ _]
      tunnel: w211 -> [_ _ _ _ _ _ _ _ _ _ _ _ _ _ _ _ w469 _ _ _ _]
      tunnel: w210 -> [_ _ _ _ _ _ _ _ _ _ _ _ _ _ _ _ w465 _ _ _ _]
      tunnel: w209 -> [w222 _ _ _ _ _ w389 _ _ _ _ _ _ _ _ _ _ _ _ _ _]
      tunnel: [w221 w266 w368 w373 w382 w386 w387 w396 w406 w413 w425 w437 w444 w447 w451 w459 w464 w486 w488 w492 w503] -> w208
      tunnel: w207 -> [w221 w266 w368 w373 w382 w386 w387 _ _ w413 w425 w437 w444 w447 w451 w459 w464 w486 w488 w492 w503]
      tunnel: w206 -> [w219 _ _ _ _ _ _ _ _ _ _ _ _ _ _ _ _ _ _ _ _]
      event Timeout {
        n125 = event-data() -> ()  [unwired: 1 in, 1 out]
        n126 = local read "Mode"() -> (w224:T4)
        n127 = case shown="\"Basic\"" "Dashboard Tab" {
          tunnel: w227 -> [_ _ w243 _ _]
          tunnel: "/TestMode/Automatic/" ("Name Pattern") -> [_ _ w242 _ _]
          tunnel: T18 [{"Operation"=enum."Clear", "Color Box"=14013909}, {"Operation"=enum."Clear", "Color Box"=14013909}, {"Operation"=enum."Clear", "Color Box"=14013909}, {"Operation"=enum."Clear", "Color Box"=14013909}, {"Operation"=enum."Update", "Color Box"=14013909}, {"Operation"=enum."Update", "Color Box"=16777215}, {"Operation"=enum."Clear", "Color Box"=14013909}, {"Operation"=enum."Clear", "Color Box"=14013909}, {"Operation"=enum."Clear", "Color Box"=14013909}] -> [_ _ w235 _ w259]
          tunnel: w224 -> [_ _ w234 _ w258]
          tunnel: u32[] [15790320, 15790320, 15790320, 15790320, 16777215, 16777215, 15790320, 15790320, 15790320] -> [_ _ _ _ w264]
          tunnel: w222 -> [_ _ _ _ w252]
          tunnel: w219 -> [_ w229 _ _ _]
          frame "Custom", Default {
          }
          frame "Basic" {
            n128 = call <vilib>:"WPI_DashboardUpdateNames.vi"("Controls on Tab"=w229) -> ()  [unwired: 11 in]
          }
          frame "Test" {
            w241 = -2 ("Active Item:Row Number")
            n129 = Index Array(array=w235, index=w234) -> (element=w236:T21)
            n130 = Unbundle(w236) -> ("Operation"=w237:enum16{"Update", "Clear"}, "Color Box"=w238:u32)
            n131 = call <vilib>:"NT Read String.vi"("Name"="/TestMode/TestName") -> ("String"=w232:string)  [unwired: 9 in, 1 out]
            n132 = call <vilib>:"NT Read and Format Entries as Tree.vi"("Operation"=w237, "Name Pattern"=w242, "Tree Refnum"=w243) -> ()  [unwired: 7 in, 2 out]
            n133 = case shown="\"\"" w232 {
              tunnel: "/TestMode/TestProgress" ("Name") -> [w245 _]
              tunnel: "/TestMode/TestProgressText" ("Name") -> [w244 _]
              frame Default {
                n134 = call <vilib>:"NT Read Number.vi"("Name"=w245) -> ("Numeric"=w246:dbl)  [unwired: 9 in, 1 out]
                n135 = call <vilib>:"NT Read String.vi"("Name"=w244) -> ("String"=w247:string)  [unwired: 9 in, 1 out]
                n136 = Bundle("Numeric"=w246, "String"=w247) -> (→"Progress":cluster{"Numeric":dbl, "String":string})  [unwired: 1 in]
              }
              frame "" {
                n137 = property on="Progress" class="Clust (strict)"("Visible"=FALSE) -> ()  [unwired: 2 in, 2 out]
                n138 = local write "Test Name"(u16 0) -> ()
              }
            }
            n139 = property on="Test Tree" class="Tree (strict)"("Active Item Row Number"=w241, "ActiveColNum"=w241, "CellBG"=w238, "Active Item Row Number"=-1 ("Active Item:Row Number"), "CellBG"=u32 5789784 ("Color Box")) -> ()  [unwired: 2 in, 2 out]
          }
          frame "Variables" {
            n140 = control-ref of="Tree"() -> (w251:refnum<vi>)
            n141 = call <vilib>:"NT Read and Format Entries as Tree.vi"("Tree Refnum"=w251) -> ()  [unwired: 9 in, 2 out]
          }
          frame "Commands" {
            w260 = u32 5789784 ("Color Box")
            w261 = T22 {"Row"=-1, "Column"=-2} ("Active Cell:Active Cell")
            w263 = T22 {"Row"=-2, "Column"=-2} ("Active Cell:Active Cell")
            n142 = Index Array(array=w264, index=w258) -> (element=w262:u32)
            n143 = Index Array(array=w259, index=w258) -> (element=w257:T21)
            n144 = Unbundle(w257) -> ("Operation"=w256:enum16{"Update", "Clear"})  [unwired: 1 out]
            n145 = local read "Command Selection"() -> (w255:i32)
            n146 = property on="Command Selection" class="MCListbox (strict)"("ActiveCell"=w263, "CellBG"=w262, "ActiveCell"=w261, "CellBG"=w260) -> ()  [unwired: 2 in, 2 out]
            n147 = call <vilib>:"WPI_DashboardUpdate RPC Info.vi"("Operation"=w256) -> ("update"=w254:bool, "commands"=w253:string[][])  [unwired: 9 in]
            n148 = property on="Command Selection" class="MCListbox (strict)"("ItemNames"=w253) -> ()  [unwired: 2 in, 2 out]
            n149 = property on="Command Params" class="Tbl (strict)"("Active Cell"=w263, "Cell BG Color"=w262, "Active Cell"=w261, "Cell BG Color"=w260) -> ()  [unwired: 2 in, 2 out]
            n150 = call <vilib>:"WPI_DashboardUpdate Command Params.vi"("Update"=w254, "NewVal"=w255, "Commands"=w253, "Param Tbl"=w252) -> ()  [unwired: 7 in, 1 out]
          }
        }
        n151 = call <vilib>:"Connextion Info.vi"() -> ("Connected"=→"NT Connection":bool)  [unwired: 10 in, 1 out]
      }
      event "Test Tree": Value Change {
        # "Show appropriate\ncontrols"
        n152 = event-data() -> ("CtlRef"=w269:refnum<vi>, "NewVal"=w267:string)  [unwired: 1 in]
        n153 = call <vilib>:"WPI_UtilitiesGetTreeIOName.vi"("NewVal"=w267, "TreeControl in"=w269) -> ("I/O Name"=w270:string)  [unwired: 9 in]
        n154 = case shown="\"Camera\"" w270 {
          selector: w270 -> [_ w277 _ w299 w308 _]
          tunnel: w267 -> [_ _ w296 w298 _ w315]
          tunnel: cluster{string[]}[] [{["640x480", "320x240", "160x120"]}, {["Auto", "Fixed indoor", "Fixed outdoor 1", "Fixed outdoor 2", "Fixed fluorescent 1", "Fixed fluorescent 2", "Hold current"]}, {["Auto", "Flicker-free 50 Hz", "Flicker-free 60 Hz", "Hold current"]}, {["None", "Prioritize frame rate", "Prioritize image quality"]}, {["Monochrome", "Color"]}] -> [_ _ _ _ _ w314]
          frame Default {
            w272 = FALSE ("Visible")
            w271 = FALSE ("Visible")
            n155 = property on="Motor" class="Clust (strict)"("Visible"=w271) -> ()  [unwired: 2 in, 2 out]
            n156 = property on="Test Ring" class="Ring (strict)"("Visible"=w271) -> ()  [unwired: 2 in, 2 out]
            n157 = property on="Rev/Fwd" class="Clust (strict)"("Visible"=w272) -> ()  [unwired: 2 in, 2 out]
            n158 = property on="On/Off" class="Bool (strict)"("Visible"=w272) -> ()  [unwired: 2 in, 2 out]
            n159 = property on="Test Slider" class="Slide (strict)"("Visible"=w272) -> ()  [unwired: 2 in, 2 out]
          }
          frame "Analog Out", "Motor", "PWM" {
            w278 = FALSE ("Visible")
            n160 = case shown="\"Analog Out\"" w277 {
              tunnel: [1.0 ("Value") -1.0 ("Value") 0.0 ("Value")] -> w276
              tunnel: [255.0 ("Value") 1.0 ("Value") 5.0 ("Value")] -> w275
              tunnel: [128.0 ("Value") 0.0 ("Value") 0.0 ("Value")] -> w274
              tunnel: [64.0 ("Value") 0.5 ("Value") 1.0 ("Value")] -> w273
              frame "PWM" {
              }
              frame "Motor", Default {
              }
              frame "Analog Out" {
              }
            }
            n161 = property on="Motor" class="Clust (strict)"("Visible"=TRUE) -> ()  [unwired: 2 in, 2 out]
            n162 = property on="Value" class="Slide (strict)"("Value"=w274, "Scale.Minimum"=w276, "Scale.Maximum"=w275, "Scale.Increment"=w273) -> ()  [unwired: 2 in, 2 out]
            n163 = property on="On/Off" class="Bool (strict)"("Visible"=w278) -> ()  [unwired: 2 in, 2 out]
            n164 = property on="Test Slider" class="Slide (strict)"("Visible"=w278) -> ()  [unwired: 2 in, 2 out]
            n165 = property on="Test Ring" class="Ring (strict)"("Visible"=w278) -> ()  [unwired: 2 in, 2 out]
            n166 = property on="Rev/Fwd" class="Clust (strict)"("Visible"=w278) -> ()  [unwired: 2 in, 2 out]
          }
          frame "Servo" {
            w294 = FALSE ("Visible")
            n167 = call <vilib>:"NT Read Number.vi"("Name"=w296) -> ("Numeric"=w295:dbl)  [unwired: 9 in, 1 out]
            n168 = property on="Test Slider" class="Slide (strict)"("Visible"=TRUE, "Scale.Maximum"=170.0 ("Scale.Range:Maximum")) -> ()  [unwired: 2 in, 2 out]
            n169 = local write "Test Slider"(w295) -> ()
            n170 = property on="Motor" class="Clust (strict)"("Visible"=w294) -> ()  [unwired: 2 in, 2 out]
            n171 = property on="Rev/Fwd" class="Clust (strict)"("Visible"=w294) -> ()  [unwired: 2 in, 2 out]
            n172 = property on="On/Off" class="Bool (strict)"("Visible"=w294) -> ()  [unwired: 2 in, 2 out]
            n173 = property on="Test Ring" class="Ring (strict)"("Visible"=w294) -> ()  [unwired: 2 in, 2 out]
          }
          frame "Relay", "Solenoid" {
            w297 = FALSE ("Visible")
            n174 = property on="Motor" class="Clust (strict)"("Visible"=w297) -> ()  [unwired: 2 in, 2 out]
            n175 = property on="Test Slider" class="Slide (strict)"("Visible"=w297) -> ()  [unwired: 2 in, 2 out]
            n176 = Search and Replace String(input string=w298, search string="/Value  **", replace string="/Direction") -> (result string=w304:string)  [unwired: 5 in, 3 out]
            n177 = property on="Test Ring" class="Ring (strict)"("Visible"=w297) -> ()  [unwired: 2 in, 2 out]
            n178 = call <vilib>:"NT Read String.vi"("Name"=w304) -> ("String"=w302:string)  [unwired: 9 in, 1 out]
            n179 = Equal?(x="Both directions", y=w302) -> (x = y?=w300:bool)
            n180 = Not(x=w300) -> (.not. x?=w301:bool)
            n181 = property on="Rev/Fwd" class="Clust (strict)"("Visible"=w300) -> ()  [unwired: 2 in, 2 out]
            n182 = property on="On/Off" class="Bool (strict)"("Visible"=w301, "Caption.Text"=w299) -> ()  [unwired: 2 in, 2 out]
          }
          frame "Compressor", "Digital Out" {
            w307 = FALSE ("Visible")
            # "Get direction and finish"
            n183 = property on="Motor" class="Clust (strict)"("Visible"=w307) -> ()  [unwired: 2 in, 2 out]
            n184 = property on="Test Slider" class="Slide (strict)"("Visible"=w307) -> ()  [unwired: 2 in, 2 out]
            n185 = property on="Test Ring" class="Ring (strict)"("Visible"=w307) -> ()  [unwired: 2 in, 2 out]
            n186 = property on="On/Off" class="Bool (strict)"("Visible"=TRUE, "Caption.Text"=w308) -> ()  [unwired: 2 in, 2 out]
            n187 = property on="Rev/Fwd" class="Clust (strict)"("Visible"=FALSE) -> ()  [unwired: 2 in, 2 out]
          }
          frame "Camera" {
            n188 = call <vilib>:"Get Last Path Segment.vi"("String in"=w315) -> ("String out"=w316:string)  [unwired: 10 in]
            n189 = property on="On/Off" class="Bool (strict)"("Visible"=FALSE) -> ()  [unwired: 2 in, 2 out]
            n190 = property on="Motor" class="Clust (strict)"("Visible"=FALSE) -> ()  [unwired: 2 in, 2 out]
            n191 = property on="Rev/Fwd" class="Clust (strict)"("Visible"=FALSE) -> ()  [unwired: 2 in, 2 out]
            n192 = case shown="\"White Balance  **\"" w316 {
              tunnel: w315 -> [w322 w331 w340 w349 w358 _ w364]
              tunnel: w314 -> [w320 w328 w337 w346 w355 _ _]
              frame "Size  **" {
                n193 = Index Array(array=w320) -> (element=w319:cluster{string[]})  [unwired: 1 in]
                n194 = call <vilib>:"NT Read String.vi"("Name"=w322) -> ("String"=w321:string)  [unwired: 9 in, 1 out]
                n195 = Unbundle(w319) -> (w317:string[])
                n196 = Match First String(2:w317, 3:w321) -> (0:w318:i32)  [unwired: 1 out]
                n197 = property on="Test Ring" class="Ring (strict)"("Value"=w318, "Strings []"=w317) -> ()  [unwired: 2 in, 2 out]
                n198 = property on="Test Ring" class="Ring (strict)"("Visible"=TRUE) -> ()  [unwired: 2 in, 2 out]
                n199 = property on="Test Slider" class="Slide (strict)"("Visible"=FALSE) -> ()  [unwired: 2 in, 2 out]
              }
              frame "White Balance  **" {
                n200 = Index Array(array=w328, index=1) -> (element=w329:cluster{string[]})
                n201 = call <vilib>:"NT Read String.vi"("Name"=w331) -> ("String"=w330:string)  [unwired: 9 in, 1 out]
                n202 = Unbundle(w329) -> (w326:string[])
                n203 = Match First String(2:w326, 3:w330) -> (0:w325:i32)  [unwired: 1 out]
                n204 = property on="Test Ring" class="Ring (strict)"("Value"=w325, "Strings []"=w326) -> ()  [unwired: 2 in, 2 out]
                n205 = property on="Test Ring" class="Ring (strict)"("Visible"=TRUE) -> ()  [unwired: 2 in, 2 out]
                n206 = property on="Test Slider" class="Slide (strict)"("Visible"=FALSE) -> ()  [unwired: 2 in, 2 out]
              }
              frame "Exposure  **" {
                n207 = Index Array(array=w337, index=2) -> (element=w338:cluster{string[]})
                n208 = call <vilib>:"NT Read String.vi"("Name"=w340) -> ("String"=w339:string)  [unwired: 9 in, 1 out]
                n209 = Unbundle(w338) -> (w334:string[])
                n210 = Match First String(2:w334, 3:w339) -> (0:w335:i32)  [unwired: 1 out]
                n211 = property on="Test Ring" class="Ring (strict)"("Value"=w335, "Strings []"=w334) -> ()  [unwired: 2 in, 2 out]
                n212 = property on="Test Ring" class="Ring (strict)"("Visible"=TRUE) -> ()  [unwired: 2 in, 2 out]
                n213 = property on="Test Slider" class="Slide (strict)"("Visible"=FALSE) -> ()  [unwired: 2 in, 2 out]
              }
              frame "Exposure Priority  **" {
                n214 = Index Array(array=w346, index=3) -> (element=w347:cluster{string[]})
                n215 = call <vilib>:"NT Read String.vi"("Name"=w349) -> ("String"=w348:string)  [unwired: 9 in, 1 out]
                n216 = Unbundle(w347) -> (w343:string[])
                n217 = Match First String(2:w343, 3:w348) -> (0:w344:i32)  [unwired: 1 out]
                n218 = property on="Test Ring" class="Ring (strict)"("Value"=w344, "Strings []"=w343) -> ()  [unwired: 2 in, 2 out]
                n219 = property on="Test Ring" class="Ring (strict)"("Visible"=TRUE) -> ()  [unwired: 2 in, 2 out]
                n220 = property on="Test Slider" class="Slide (strict)"("Visible"=FALSE) -> ()  [unwired: 2 in, 2 out]
              }
              frame "Color Enable  **" {
                n221 = Index Array(array=w355, index=4) -> (element=w356:cluster{string[]})
                n222 = call <vilib>:"NT Read String.vi"("Name"=w358) -> ("String"=w357:string)  [unwired: 9 in, 1 out]
                n223 = Unbundle(w356) -> (w352:string[])
                n224 = Match First String(2:w352, 3:w357) -> (0:w353:i32)  [unwired: 1 out]
                n225 = property on="Test Ring" class="Ring (strict)"("Value"=w353, "Strings []"=w352) -> ()  [unwired: 2 in, 2 out]
                n226 = property on="Test Ring" class="Ring (strict)"("Visible"=TRUE) -> ()  [unwired: 2 in, 2 out]
                n227 = property on="Test Slider" class="Slide (strict)"("Visible"=FALSE) -> ()  [unwired: 2 in, 2 out]
              }
              frame Default {
                n228 = property on="Test Ring" class="Ring (strict)"("Visible"=FALSE) -> ()  [unwired: 2 in, 2 out]
                n229 = property on="Test Slider" class="Slide (strict)"("Visible"=FALSE) -> ()  [unwired: 2 in, 2 out]
              }
              frame "Brightness  **", "Color Level  **", "Compression  **", "FPS  **", "Sharpness  **" {
                n230 = call <vilib>:"NT Read Number.vi"("Name"=w364) -> ("Numeric"=w363:dbl)  [unwired: 9 in, 1 out]
                n231 = local write "Test Slider"(w363) -> ()
                n232 = property on="Test Slider" class="Slide (strict)"("Visible"=TRUE, "Scale.Maximum"=100.0 ("Scale.Range:Maximum")) -> ()  [unwired: 2 in, 2 out]
                n233 = property on="Test Ring" class="Ring (strict)"("Visible"=FALSE) -> ()  [unwired: 2 in, 2 out]
              }
            }
          }
        }
        n234 = property on="Progress" class="Clust (strict)"("Visible"=FALSE) -> ()  [unwired: 2 in, 2 out]
      }
      event "Test Name": Mouse Enter {
        # "Populate the ring with the list of tests"
        n235 = event-data() -> ()  [unwired: 1 in, 1 out]
        n236 = call <vilib>:"NT Read String Array.vi"("Name"="/TestMode/TestList") -> ("String Array"=w372:string[])  [unwired: 9 in, 1 out]
        n237 = Build Array (concatenate)("Select the test to run...", w372) -> (w371:string[])
        n238 = property on="Test Name" class="Ring (strict)"("Strings []"=w371) -> ()  [unwired: 2 in, 2 out]
      }
      event "Test Name": Value Change {
        w374 = FALSE ("Visible")
        # "Tell the robot the test name to run"
        n239 = event-data() -> ("NewVal"=w378:u16)  [unwired: 1 in]
        n240 = property on="Test Name" class="Ring (strict)"() -> ("Strings []"=w379:string[])  [unwired: 2 in, 2 out]
        n241 = local write "Progress"(T6 {"Test Progress"=0, "Test Progress Text"=""} ("Progress")) -> ()
        n242 = Index Array(array=w379, index=w378) -> (element=w377:string)
        n243 = call <vilib>:"NT Write String.vi"("String"=w377, "Name"="/TestMode/TestName") -> ()  [unwired: 9 in, 1 out]
        n244 = property on="Progress" class="Clust (strict)"("Visible"=TRUE) -> ()  [unwired: 2 in, 2 out]
        n245 = property on="Motor" class="Clust (strict)"("Visible"=w374) -> ()  [unwired: 2 in, 2 out]
        n246 = property on="Test Slider" class="Slide (strict)"("Visible"=w374) -> ()  [unwired: 2 in, 2 out]
        n247 = property on="On/Off" class="Bool (strict)"("Visible"=w374) -> ()  [unwired: 2 in, 2 out]
        n248 = property on="Rev/Fwd" class="Clust (strict)"("Visible"=w374) -> ()  [unwired: 2 in, 2 out]
        n249 = property on="Test Ring" class="Ring (strict)"("Visible"=w374) -> ()  [unwired: 2 in, 2 out]
      }
      event "Select Auto": Mouse Enter {
        # "Populate the combo box with the list of autonomous options"
        n250 = event-data() -> ()  [unwired: 1 in, 1 out]
        n251 = call <vilib>:"NT Read String Array.vi"("Name"="Auto List") -> ("String Array"=w381:string[])  [unwired: 9 in, 1 out]
        n252 = property on="Select Auto" class="CmbBox"("Strings[]"=w381) -> ()  [unwired: 2 in, 2 out]
      }
      event "Select Auto": Value Change {
        # "User modified the Auto Selection. Write to NT variable so robot knows."
        n253 = event-data() -> ("NewVal"=w384:string)  [unwired: 1 in]
        n254 = call <vilib>:"NT Write String.vi"("String"=w384, "Name"="Auto Selector") -> ()  [unwired: 9 in, 1 out]
      }
      event "Command Selection": Value Change {
        # "Get the params and show in table"
        n255 = event-data() -> ("NewVal"=w390:i32)  [unwired: 1 in]
        n256 = property on="Command Selection" class="MCListbox (strict)"() -> ("ItemNames"=w388:string[][])  [unwired: 2 in, 2 out]
        n257 = call <vilib>:"WPI_DashboardUpdate Command Params.vi"("NewVal"=w390, "Commands"=w388, "Param Tbl"=w389) -> ()  [unwired: 8 in, 1 out]
      }
      event "Execute Command": Value Change {
        # "Started one, Unique ID holds\nresponse"
        n258 = event-data() -> ()  [unwired: 1 in, 1 out]
        n259 = property on="Command Selection" class="MCListbox (strict)"() -> ("ItemNames"=w401:string[][])  [unwired: 2 in, 2 out]
        n260 = Index Array(array=w401, index (row)="Command Selection", index (col)=0) -> (element=w399:string)
        n261 = call <vilib>:"Invoke Commands.vi"("Command Params"="Command Params", "Function Name"=w399) -> ("Params"=w395:u8, "Started"=w394:bool)  [unwired: 7 in, 1 out]
        n262 = Array Subset(array="Command Params", length (row)=w395) -> (w396:string[][])  [unwired: 3 in]
        n263 = Select(t="Executing" ("Cmd Status"), s=w394, f="" ("Cmd Status")) -> (s? t:f=→"Cmd Status":string)
      }
      event "Command Selection": Double Click {
        n264 = event-data() -> ("Row"=w409:i32)  [unwired: 1 in]
        n265 = property on="Command Selection" class="MCListbox (strict)"() -> ("ItemNames"=w412:string[][])  [unwired: 2 in, 2 out]
        n266 = local read "Command Params"() -> (w408:string[][])
        n267 = Index Array(array=w412, index (row)=w409, index (col)=0) -> (element=w410:string)
        n268 = call <vilib>:"Invoke Commands.vi"("Command Params"=w408, "Function Name"=w410) -> ("Params"=w407:u8, "Started"=w402:bool)  [unwired: 7 in, 1 out]
        n269 = Array Subset(array=w408, length (row)=w407) -> (w406:string[][])  [unwired: 3 in]
        n270 = Select(t="Executing" ("Cmd Status"), s=w402, f="" ("Cmd Status")) -> (s? t:f=w403:string)
        n271 = local write "Cmd Status"(w403) -> ()
      }
      event "CheckList": Double Click {
        # "Shift clears all"
        # "Update symbols on the listbox"
        n272 = event-data() -> ("PlatMods.Shift"=w414:bool, "Row"=w416:i32)  [unwired: 1 in]
        n273 = case shown="True" w414 {
          tunnel: w416 -> [w420 _]
          tunnel: 1 -> [w419 _]
          frame False {
            n274 = property on="CheckList" class="LstBox (strict)"() -> ("Item Symbols"=w418:i32[])  [unwired: 2 in, 2 out]
            n275 = Replace Array Subset(array=w418, new element=w419, index=w420) -> (w417:i32[])
            n276 = property on="CheckList" class="LstBox (strict)"("Item Symbols"=w417) -> ()  [unwired: 2 in, 2 out]
          }
          frame True {
            w421 = 0 ("Top Row")
            n277 = property on="CheckList" class="LstBox (strict)"() -> ("Number of Rows"=w423:u32)  [unwired: 2 in, 2 out]
            n278 = Initialize Array(0, w423) -> (w422:i32[])
            n279 = property on="CheckList" class="LstBox (strict)"("Top Row"=w421, "Value"=w421, "Item Symbols"=w422) -> ()  [unwired: 2 in, 2 out]
          }
        }
      }
      event "CheckList": Key Down {
        # "Update symbols on the listbox\nLeft and right keys check and uncheck"
        n280 = event-data() -> ("VKey"=w427:T19)  [unwired: 1 in]
        n281 = case shown="\"Left\", \"Right\"" w427 {
          selector: w427 -> [w432 _]
          tunnel: eventvkey."Left" ("VKey") -> [w430 _]
          frame "Left", "Right" {
            n282 = Equal?(x=w430, y=w432) -> (x = y?=w431:bool)
            n283 = Select(t=0, s=w431, f=1) -> (s? t:f=w433:i32)
            n284 = property on="CheckList" class="LstBox (strict)"() -> ("Item Symbols"=w436:i32[])  [unwired: 2 in, 2 out]
            n285 = Replace Array Subset(array=w436, new element=w433, index="CheckList") -> (w435:i32[])
            n286 = property on="CheckList" class="LstBox (strict)"("Item Symbols"=w435) -> ()  [unwired: 2 in, 2 out]
          }
          frame Default {
          }
        }
      }
      event "Motor.Enable": Value Change {
        # "When the test mode otor enable helper is set, update that\ntree row item's value"
        n287 = event-data() -> ("NewVal"=w442:bool)  [unwired: 1 in]
        n288 = Unbundle("Motor") -> ("Value"=w441:dbl)  [unwired: 1 out]
        n289 = Select(t=w441, s=w442, f=0.0) -> (s? t:f=w439:dbl)
        n290 = call <vilib>:"NT Write Number.vi"("Numeric"=w439, "Name"=w438) -> ()  [unwired: 9 in, 1 out]
      }
      event "Test Slider": Value Change {
        # "When the test mode slider helper is set, update that\ntree row item's value"
        n291 = event-data() -> ("NewVal"=w445:dbl)  [unwired: 1 in]
        n292 = call <vilib>:"NT Write Number.vi"("Numeric"=w445, "Name"=w446) -> ()  [unwired: 9 in, 1 out]
      }
      event "On/Off": Value Change {
        # "When the test mode on/off helper value is set, update that\ntree row item's value"
        n293 = event-data() -> ("NewVal"=w450:bool)  [unwired: 1 in]
        n294 = Boolean To (0,1)(Boolean=w450) -> (0, 1=w449:i16)
        n295 = call <vilib>:"NT Write Number.vi"("Numeric"=w449, "Name"=w448) -> ()  [unwired: 9 in, 1 out]
      }
      event "Rev/Fwd": Value Change {
        # "When the test mode helper value for relays is set, update that\ntree row item's value"
        n296 = event-data() -> ("NewVal.Forward"=w458:bool, "NewVal.Reverse"=w457:bool)  [unwired: 1 in]
        n297 = Boolean To (0,1)(Boolean=w458) -> (0, 1=w454:i16)
        n298 = Boolean To (0,1)(Boolean=w457) -> (0, 1=w456:i16)
        n299 = Negate(x=w456) -> (-x=w455:i16)
        n300 = Add(x=w454, y=w455) -> (x+y=w453:i16)
        n301 = call <vilib>:"NT Write Number.vi"("Numeric"=w453, "Name"=w452) -> ()  [unwired: 9 in, 1 out]
      }
      event "Test Ring": Value Change {
        # "When a test mode helper value is selected from the ring,\nset the tree item's variable to the string value"
        n302 = event-data() -> ("NewVal"=w462:u16)  [unwired: 1 in]
        n303 = property on="Test Ring" class="Ring (strict)"() -> ("Strings []"=w463:string[])  [unwired: 2 in, 2 out]
        n304 = Index Array(array=w463, index=w462) -> (element=w461:string)
        n305 = call <vilib>:"NT Write String.vi"("String"=w461, "Name"=w460) -> ()  [unwired: 9 in, 1 out]
      }
      event "Rec Mode": Value Change {
        # "Update globals for recording mode and path to read log from.\nClear when logging and let NetworkTables set path for vision to\nuse."
        n306 = event-data() -> ("NewVal"=w474:enum32{"Stop", "Record", "Playback"})  [unwired: 1 in]
        n307 = global write "WPI_DashboardLogging Global.vi" "Logging Filename"(path "") -> ()
        n308 = global write "WPI_DashboardLogging Global.vi" "Recording"(w474) -> ()
        n309 = case shown="\"Playback\"" w474 {
          tunnel: w473 -> [_ w476 w485]
          tunnel: [_ _ w484] -> w471
          tunnel: [_ _ w483] -> _
          tunnel: w469 -> [_ _ w481]
          tunnel: cluster{i32, i32} {-250, 170} -> [_ _ w480]
          tunnel: [_ _ T20 {"Image Size"=TRUE, "Image Type"=TRUE, "Pixel Value"=TRUE, "ROI Information"=TRUE, "Zoom Factor"=FALSE} ("Image Information Shown:All Elements")] -> w467
          tunnel: [_ _ TRUE ("Zoom Factor")] -> w466
          tunnel: w465 -> [_ _ w477]
          frame Default {
          }
          frame "Stop", "Record" {
            # "Place Window too"
            n310 = invoke class="VI" method="FP.Close"(reference=w476) -> (reference out=w475:refnum<vi>)  [unwired: 2 in, 2 out]
            n311 = invoke class="VI" method="Abort VI"(reference=w475) -> ()  [unwired: 2 in, 3 out]
          }
          frame "Playback" {
            n312 = call "Open Playback Panel.vi"("Offset"=w480, "DB VI Ref"=w481, "Playback in"=w485) -> ("Playback out"=w482:refnum<vi>)  [unwired: 8 in]
            n313 = register-events(w482, w477) -> (reference out=w484:refnum<event-registration>, error out=w483:errorcluster)  [unwired: 2 in]
          }
        }
        n314 = property on="Camera Image" class="ImageControl"("Image Information Shown"=w467, "Image Information Visible"=w466) -> ()  [unwired: 2 in, 2 out]
        n315 = call <vilib>:"WPI_DashboardNT Log FieldName Cache.vi"("Operation"=enum16{"Lookup/Add", "Index", "Clear"}."Clear") -> ()  [unwired: 8 in, 3 out]
      }
      event Panel Close {
        w487 = enum32{"Stop", "Record", "Playback"}."Stop" ("Rec Mode")
        # "Playback window has been closed, abort"
        n316 = event-data() -> ()  [unwired: 1 in, 4 out]
        n317 = local write "Rec Mode"(w487) -> ()
        n318 = global write "WPI_DashboardLogging Global.vi" "Recording"(w487) -> ()
      }
      event Panel Close {
        # "Abort playback window and ourself"
        n319 = event-data() -> ()  [unwired: 1 in, 4 out]
        n320 = invoke class="VI" method="FP.Close"(reference=w491) -> (reference out=w490:refnum<vi>)  [unwired: 2 in, 2 out]
        n321 = invoke class="VI" method="Abort VI"(reference=w490) -> (error out=w489:errorcluster)  [unwired: 2 in, 2 out]
        n322 = invoke class="VI" method="Abort VI"(error in=w489) -> ()  [unwired: 2 in, 3 out]
      }
      event User Event {
        n323 = event-data() -> ("IDs"=w498:cluster{"RPC field ID":u16, "Unique ID":u16}, "String"=w497:string)  [unwired: 1 in]
        n324 = Bundle("IDs"=w498, "String"=w497) -> (w496:T8)  [unwired: 1 in]
        n325 = call <vilib>:"Retrieve RPC Response.vi"("RPC Response"=w496) -> ("Output"=w494:string[][])  [unwired: 10 in]
        n326 = Build Array (concatenate)(w492, w494) -> (w493:string[][])
        n327 = local write "Command Params"(w493) -> ()
        n328 = local write "Cmd Status"("" ("Cmd Status")) -> ()
      }
      event "Tree": Double Click {
        n329 = event-data() -> ("PlatMods"=w502:T23, "Tag"=w501:string)  [unwired: 1 in]
        n330 = Unbundle(w502) -> ("Shift"=w500:bool)  [unwired: 4 out]
        n331 = Not(x=w500) -> (.not. x?=w499:bool)
        n332 = call <vilib>:"NT Update Persistence.vi"("Persistence"=w499, "Name"=w501) -> ()  [unwired: 9 in, 1 out]
      }
    }
  }
  n333 = while {
    tunnel: w64 -> [w505]
    i -> [w508]
    stop <- FALSE stop-if-true
    n334 = Wait (ms)(milliseconds to wait=u32 100) -> ()  [unwired: 1 out]
    n335 = case shown="\"Playback\"" "Rec Mode" {
      tunnel: w508 -> [_ _ w523]
      tunnel: [u32 2829099 ("Base Color") u32 11141120 ("Target Color") w512] -> w504
      frame "Stop", Default {
        # "Reset the color, extra updates don't cost much"
      }
      frame "Record" {
      }
      frame "Playback" {
        # "Playback"
        n336 = Quotient & Remainder(x=w523, y=u32 50 ("milliseconds to wait")) -> (x-y*floor(x/y)=w519:u32)  [unwired: 1 out]
        n337 = Divide(x=w519, y=u32 50 ("milliseconds to wait")) -> (x/y=w516:dbl)
        n338 = Multiply(x=6.283185307179586, y=w516) -> (x*y=w521:dbl)
        n339 = Sine(x=w521) -> (sin(x)=w520:dbl)
        n340 = Absolute Value(x=w520) -> (abs(x)=w513:dbl)
        n341 = call "Interpolate RGB Color.vi"("Proportion"=w513, "Target Color"=u32 30976, "Base Color"=u32 2829099) -> ("Result Color"=w512:u32)  [unwired: 8 in]
      }
    }
    n342 = property class="Pane"(reference=w505, "PaneColor"=w504) -> ()  [unwired: 1 in, 2 out]
  }
  n343 = local write "Dashboard Tab"(T2."Drive" ("Dashboard Tab")) -> ()
  n344 = property on="On/Off" class="Bool (strict)"("Visible"=w33) -> ()  [unwired: 2 in, 2 out]
  n345 = property on="Motor" class="Clust (strict)"("Visible"=w33) -> ()  [unwired: 2 in, 2 out]
  n346 = property on="Progress" class="Clust (strict)"("Visible"=w33) -> ()  [unwired: 2 in, 2 out]
  n347 = property on="Test Ring" class="Ring (strict)"("Visible"=w33) -> ()  [unwired: 2 in, 2 out]
  n348 = property on="Rev/Fwd" class="Clust (strict)"("Visible"=w33) -> ()  [unwired: 2 in, 2 out]
  n349 = while {
    tunnel: u16 1741 ("timeout ms (25000)") -> [w525]
    stop <- FALSE stop-if-true
    n350 = TCP Create Listener(10:w525) -> (0:w524:errorcluster, 3:w526:refnum<k5>)  [unwired: 4 in, 1 out]
    n351 = case shown="No Error" w524 {
      selector: w524 -> [w528 _]
      tunnel: w526 -> [w529 _]
      frame No Error {
        n352 = while {
          tunnel: w529 -> [w532]
          tunnel: w528 -> [w531]
          stop <- FALSE stop-if-true
          n353 = TCP Wait On Listener(8:w531, 11:w532) -> (0:w533:errorcluster, 4:w534:refnum<k5>)  [unwired: 2 in, 3 out]
          n354 = local write "TCP"(w534) -> ()
          n355 = case shown="No Error" w533 {
            frame No Error {
            }
            frame Error {
              n356 = Wait (ms)(milliseconds to wait=u32 1000) -> ()  [unwired: 1 out]
            }
          }
        }
      }
      frame Error {
        n357 = Wait (ms)(milliseconds to wait=u32 1000) -> ()  [unwired: 1 out]
      }
    }
  }
  n358 = local write "Command Selection"(u16 0 ("milliseconds to wait")) -> ()
  n359 = local write "Command Params"(string[][] [] ("Command Params")) -> ()
  n360 = global write "WPI_DashboardLogging Global.vi" "Recording"(w58) -> ()
  n361 = local write "Rec Mode"(w58) -> ()
  n362 = call <vilib>:"NT Write String.vi"("String"="Select Auto", "Name"="Auto Selector") -> ()  [unwired: 9 in, 1 out]
